vi "Translator.File.Read.FP.vi"(8 "error in":errorcluster, 9 "font name":string, 10 "Translation file":path=path "D:/PL_0125_Sapphire_Automation_branches/SOFTWARE_v1.1-Translation/settings/Translation-Chinese.ini", 11 "VI ref in [ ]":refnum<vi>[](array[refnum])) -> (0 "error out":errorcluster, 3 "VI ref out [ ]":refnum<vi>[](array[refnum]))   [LabVIEW 2019, in "Tools.lvlib"]
uses:
  Tools.lvlib
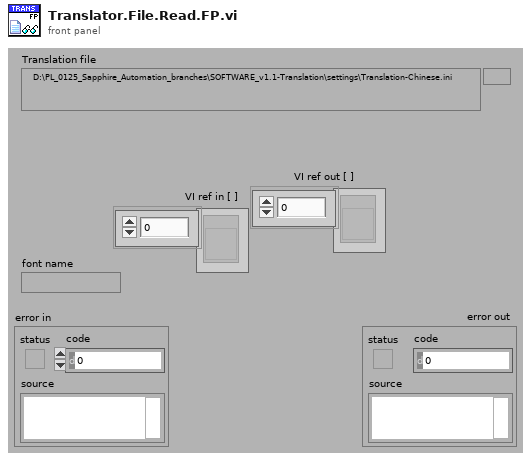
[diagram p1: front panel]
types:
  T1 = typedef "Tools.lvlib/Translator.ControlData.ctl" = cluster{"ref":refnum<vi>, "strict?":bool, "ignore?":bool, "type":T2, "root":string, "label":string, "caption":string, "bln.false":string, "bln.true":string, "cols":string[], "rows":string[]}
  T2 = typedef "Tools.lvlib/Translator.ControlTypes.ctl" = enum16{"Cluster", "Array", "Boolean", "Ring", "String", "Tab", "Listbox", "Multicolumn listbox", "Table", "Other"}
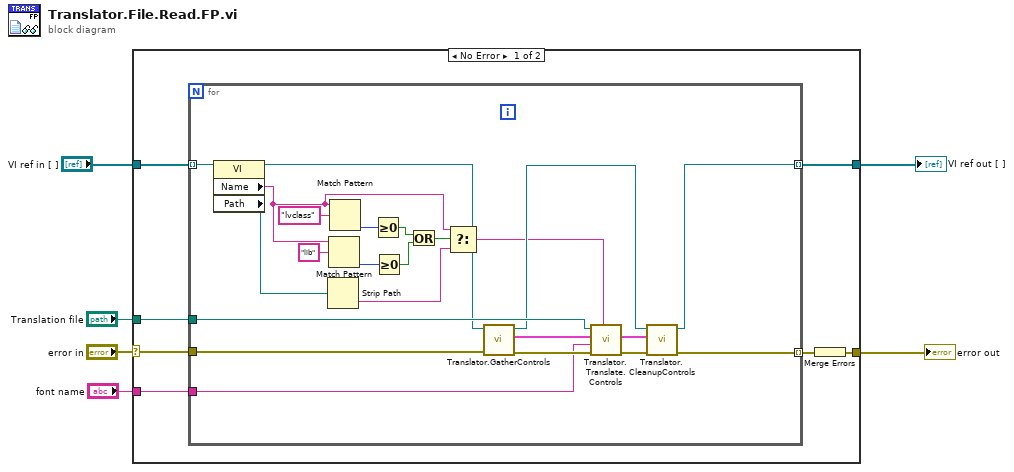
[diagram p0: block diagram]
diagram:
  n1 = case shown="No Error" "error in" {
    selector: "error in" -> [w12 w37]
    tunnel: "Translation file" -> [w10 _]
    tunnel: [w8 w37] -> w5
    tunnel: "VI ref in [ ]" -> [w9 w36]
    tunnel: "font name" -> [w13 _]
    tunnel: [w7 w36] -> w1
    frame No Error {
      n2 = for {
        tunnel: w9 -> [w30] mode=indexing
        tunnel: w13 -> [w34]
        tunnel: w10 -> [w32]
        tunnel: w12 -> [w27]
        tunnel: [w25] -> w11 mode=indexing
        tunnel: [w26] -> w7 mode=indexing
        n3 = property class="VI"(reference=w30) -> (reference out=w29:refnum<vi>, "Name"=w16:string, "Path"=w15:path)  [unwired: 1 in, 1 out]
        n4 = Strip Path(path=w15) -> (name=w14:string)  [unwired: 1 out]
        n5 = Match Pattern(string=w16, regular expression="lib") -> (offset past match=w21:i32)  [unwired: 1 in, 3 out]
        n6 = Match Pattern(string=w16, regular expression="lvclass") -> (offset past match=w22:i32)  [unwired: 1 in, 3 out]
        n7 = Greater Or Equal To 0?(x=w22) -> (x >= 0?=w19:bool)
        n8 = Greater Or Equal To 0?(x=w21) -> (x >= 0?=w20:bool)
        n9 = Or(x=w19, y=w20) -> (x .or. y?=w18:bool)
        n10 = Select(t=w16, s=w18, f=w14) -> (s? t:f=w17:string)
        n11 = call "Translator.GatherControls.vi"("error in"=w27, "VI ref in"=w29) -> ("error out"=w35:errorcluster, "Controls out"=w31:T1[], "VI ref out"=w28:refnum<vi>)  [unwired: 7 in]
        n12 = call "Translator.Translate.Controls.vi"("group"=w17, "error in"=w35, "font name"=w34, "Controls out"=w31, "Translation file"=w32) -> ("error out"=w33:errorcluster)  [unwired: 6 in]
        n13 = call "Translator.CleanupControls.vi"("error in"=w33, "Controls"=w31, "VI ref in"=w28) -> ("error out"=w25:errorcluster, "VI ref out"=w26:refnum<vi>)  [unwired: 7 in]
      }
      n14 = Merge Errors(w11) -> (w8:errorcluster)
    }
    frame Error {
    }
  }
  "error out" <- w5
  "VI ref out [ ]" <- w1
